vi "PowerModeSwitch.vi"(8 "error in (no error)":errorcluster, 11 "Data Cluster In":T1 {"VestaTemperature"."Water Heater Temp (°F)" min=32 max=203}) -> (0 "error out":errorcluster, 3 "Data Cluster out":T1 {"VestaTemperature"."Water Heater Temp (°F)" min=32 max=203}, 4 "Send_Vesta_Message":u8, 6 "Send_Timer_Message":u8)   [LabVIEW 2023]
uses:
  Drivers/Resideo Gas Valve/Type Definitions/Vesta Info.ctl
  Drivers/Resideo Gas Valve/Type Definitions/Temperature Control.ctl
  controls/Burner Duty Cycle.ctl
  controls/Timer Application Cluster.ctl
  controls/UI Data.ctl
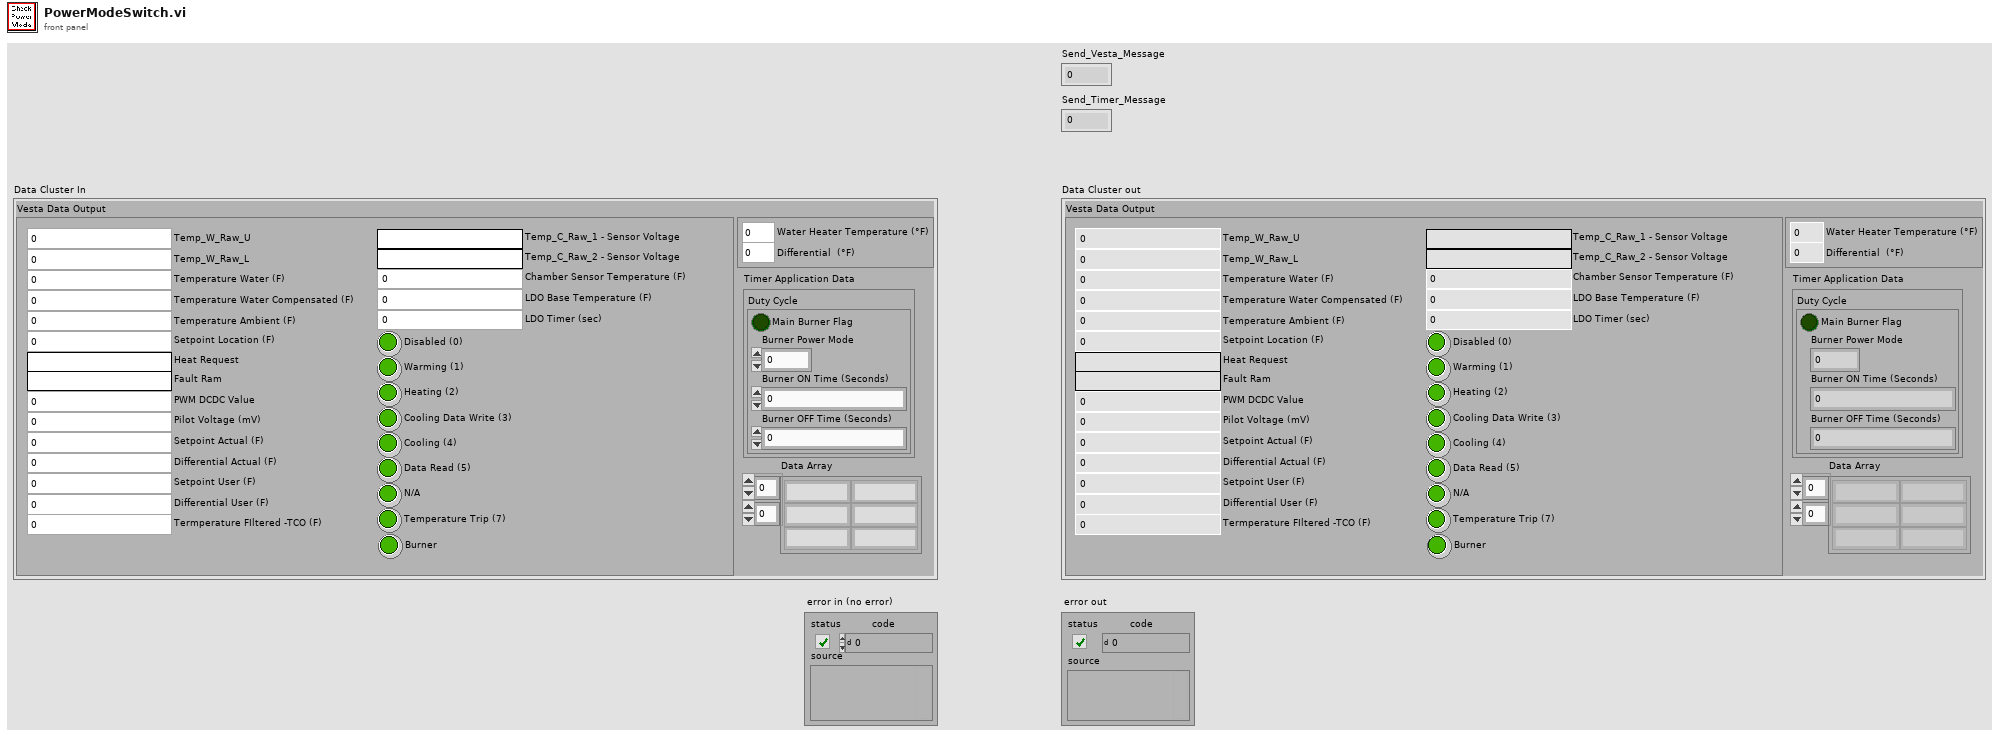
[diagram p1: front panel]
types:
  T1 = typedef "UI Data.ctl" = cluster{"Vesta Data Output":T2, "VestaTemperature":T3, "Timer Application Data":T4, "Data Array":string[][]}
  T2 = typedef "Vesta Info.ctl" = cluster{"Temp_W_Raw_U":u16, "Temp_W_Raw_L":u16, "Temperature Water (F)":dbl, "Temperature Water Compensated (F)":dbl, "Temperature Ambient (F)":dbl, "Setpoint Location (F)":dbl, "Heat Request":string, "Fault Ram":string, "PWM DCDC Value":u16, "Pilot Voltage (mV)":dbl, "Setpoint Actual (F)":dbl, "Differential Actual (F)":dbl, "Setpoint User (F)":dbl, "Differential User (F)":dbl, "Termperature FIltered -TCO (F)":dbl, "Temp_C_Raw_1 - Sensor Voltage":string, "Temp_C_Raw_2 - Sensor Voltage":string, "Chamber Sensor Temperature (F)":dbl, "LDO Base Temperature (F)":dbl, "LDO Timer (sec)":i16, "Disabled (0)":bool, "Warming (1)":bool, "Heating (2)":bool, "Cooling Data Write (3)":bool, "Cooling (4)":bool, "Data Read (5)":bool, "N/A":bool, "Temperature Trip (7)":bool, "Burner":bool}
  T3 = typedef "Temperature Control.ctl" = cluster{"Water Heater Temp (°F)":u16, "Differential  (°F)":dbl}
  T4 = typedef "Timer Application Cluster.ctl" = cluster{"Duty Cycle":T5}
  T5 = typedef "Burner Duty Cycle.ctl" = cluster{"Burner ON Time (Seconds)":dbl, "Burner OFF Time (Seconds)":dbl, "Main Burner Flag":bool, "Burner Power Mode":u8}
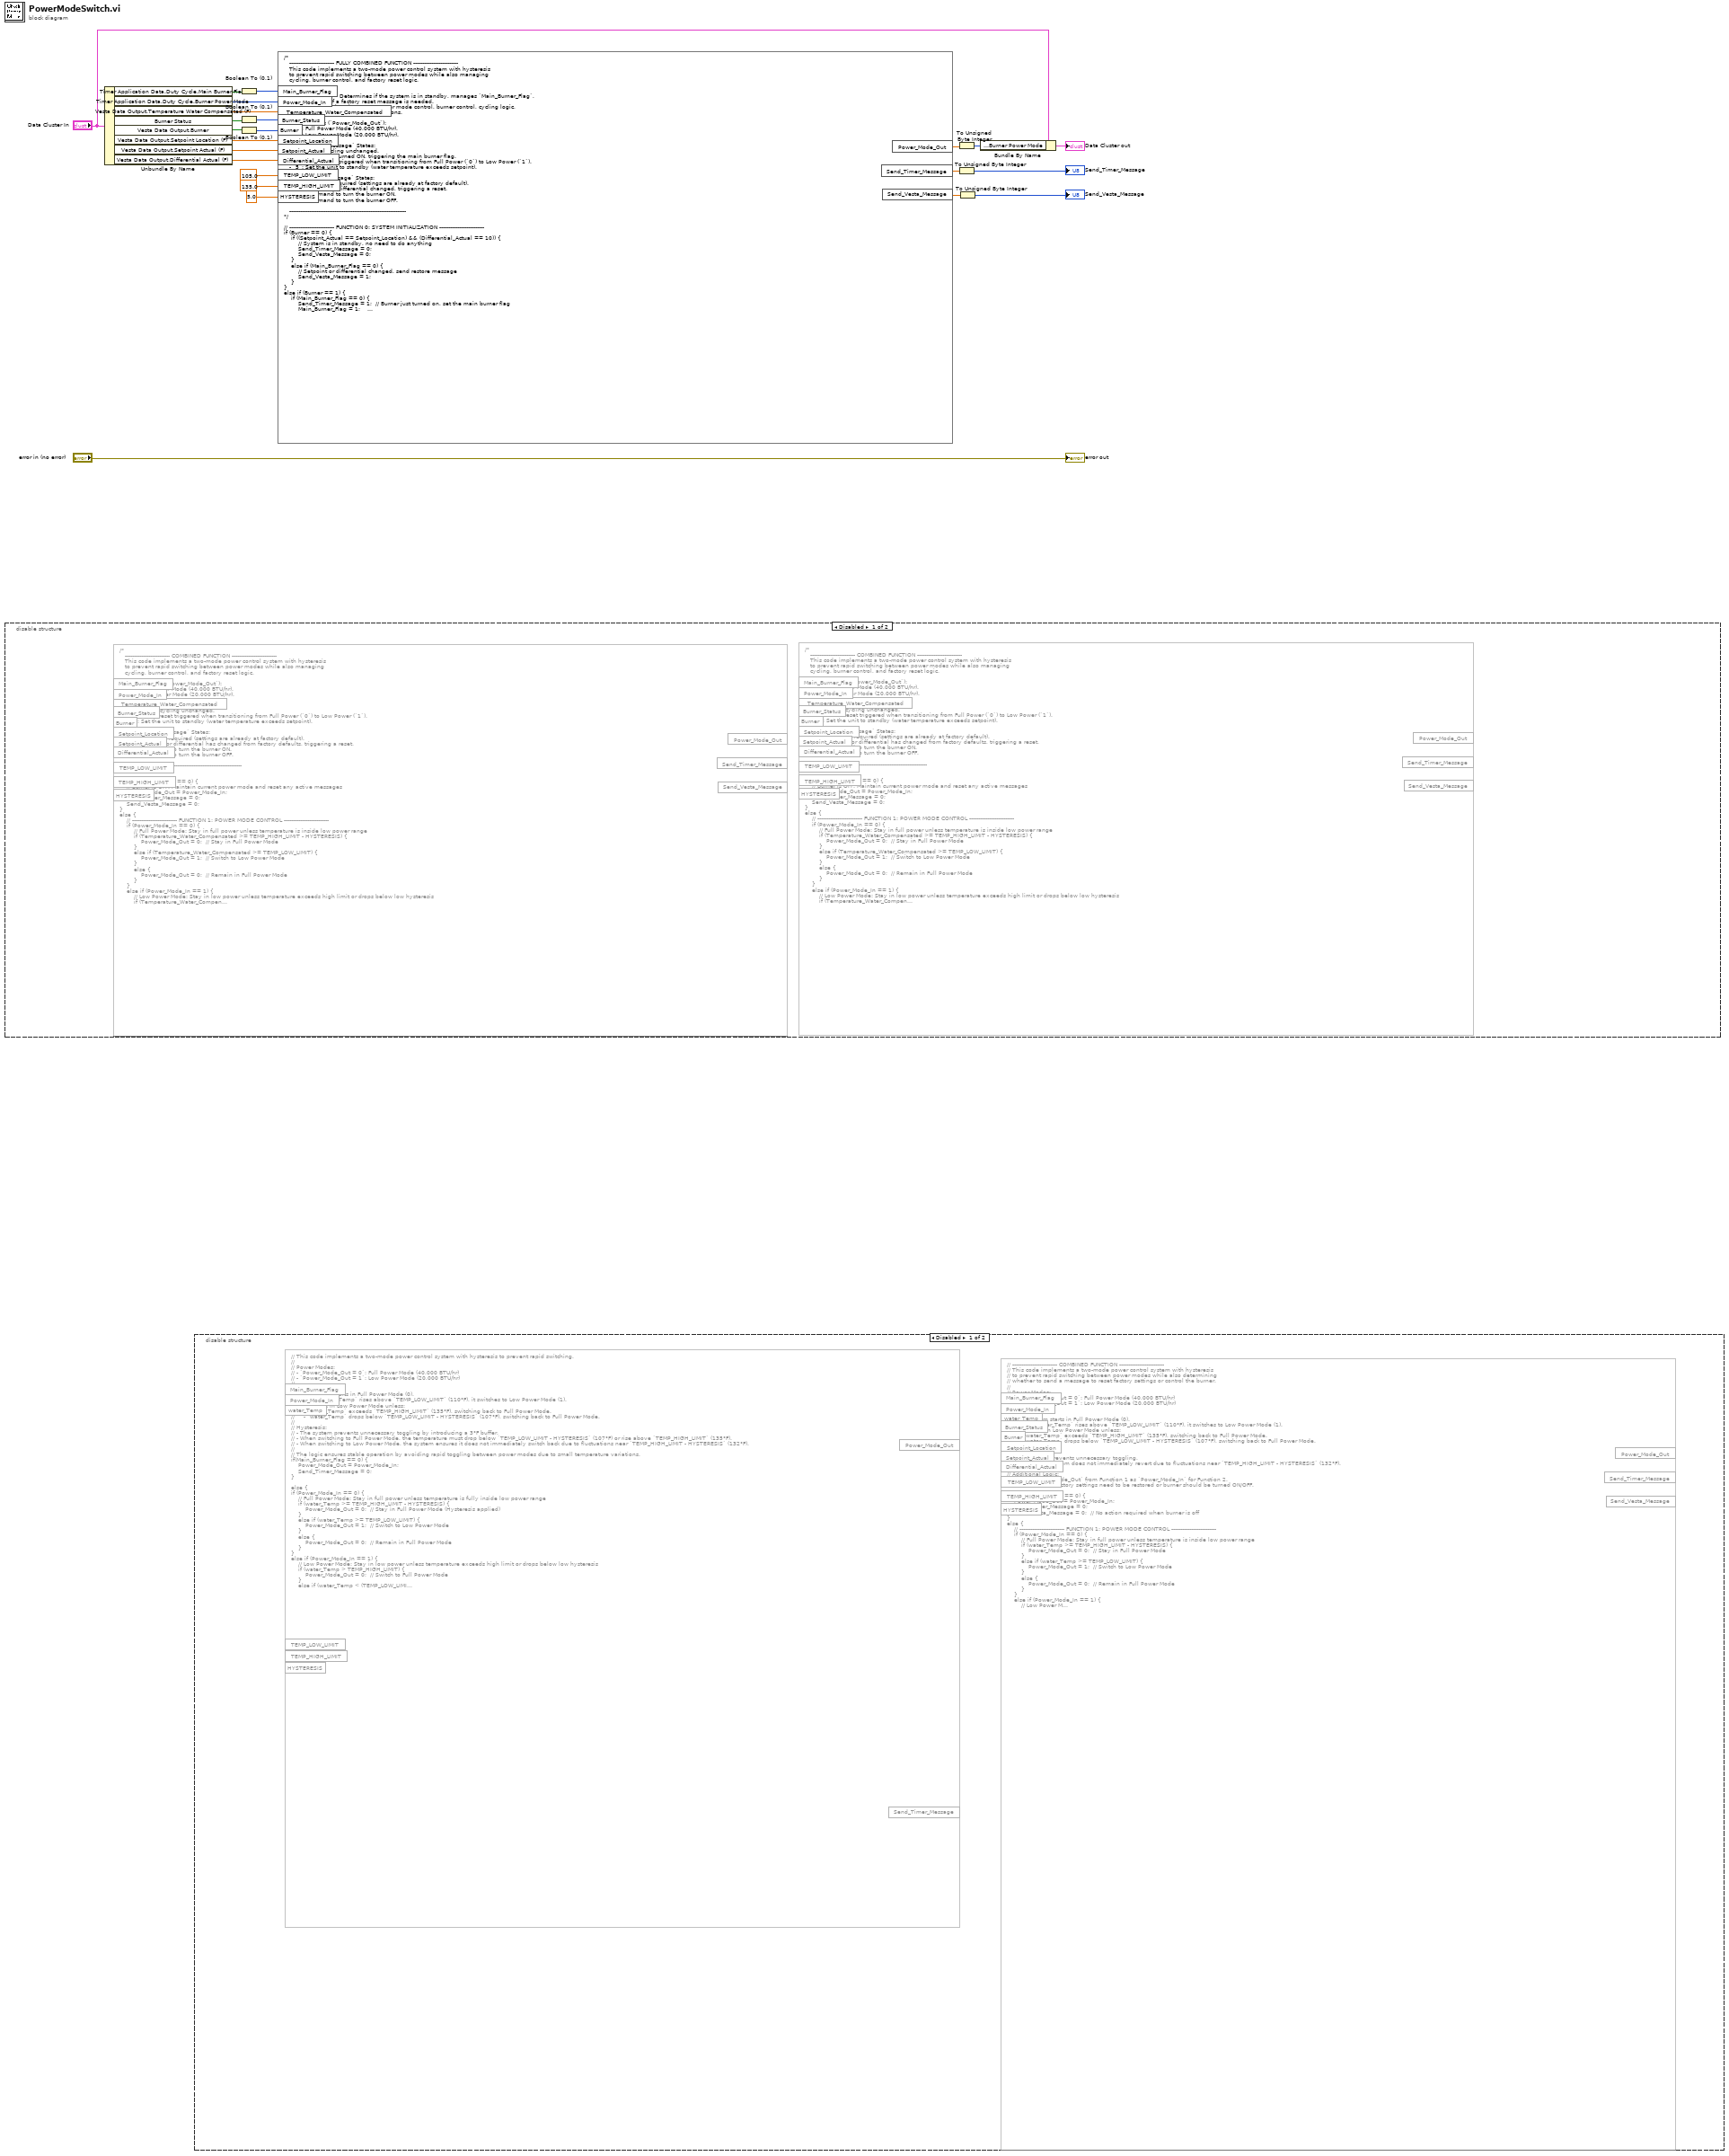
[diagram p0: block diagram]
diagram:
  n1 = disable-structure shown="Disabled" {
    frame Disabled {
      n2 = formula code="/*  \n   ------------------------- COMBINED FUNCTION -------------------------  \n   This code implements a two-mode power control system with hysteresis  \n   to prevent rapid switching between power modes while also managing  \n   cycling, burner control, and factory reset logic.\n\n   Power Modes (`Power_Mode_Out`):  \n   - `0`: Full Power Mode (40,000 BTU/hr).  \n   - `1`: Low Power Mode (20,000 BTU/hr).  \n\n   `Send_Timer_Message` States:  \n   - `0`: Leave cycling unchanged.  \n   - `2`: Timer reset triggered when transitioning from Full Power (`0`) to Low Power (`1`).  \n   - `5`: Set the unit to standby (water temperature exceeds setpoint).  \n\n   `Send_Vesta_Message` States:  \n   - `0`: No action required (settings are already at factory default).  \n   - `1`: Setpoint or differential has changed from factory defaults, triggering a reset.  \n   - `2`: Command to turn the burner ON.  \n   - `3`: Command to turn the burner OFF.  \n\n   -----------------------------------------------------------------\n*/\n\nif (Main_Burner_Flag == 0) {\n    // Burner is OFF: Maintain current power mode and reset any active messages\n    Power_Mode_Out = Power_Mode_In;\n    Send_Timer_Message = 0;\n    Send_Vesta_Message = 0;\n} \nelse {\n    // ------------------------- FUNCTION 1: POWER MODE CONTROL -------------------------\n    if (Power_Mode_In == 0) { \n        // Full Power Mode: Stay in full power unless temperature is inside low power range\n        if (Temperature_Water_Compensated >= TEMP_HIGH_LIMIT - HYSTERESIS) {\n            Power_Mode_Out = 0;  // Stay in Full Power Mode\n        } \n        else if (Temperature_Water_Compensated >= TEMP_LOW_LIMIT) {\n            Power_Mode_Out = 1;  // Switch to Low Power Mode\n        } \n        else {\n            Power_Mode_Out = 0;  // Remain in Full Power Mode\n        }\n    } \n    else if (Power_Mode_In == 1) { \n        // Low Power Mode: Stay in low power unless temperature exceeds high limit or drops below low hysteresis\n        if (Temperature_Water_Compensated > TEMP_HIGH_LIMIT) {\n            Power_Mode_Out = 0;  // Switch to Full Power Mode\n        } \n        else if (Temperature_Water_Compensated < (TEMP_LOW_LIMIT - HYSTERESIS)) {\n            Power_Mode_Out = 0;  // Switch to Full Power Mode\n        } \n        else {\n            Power_Mode_Out = 1;  // Stay in Low Power Mode\n        }\n    }\n\n    // Check if low power mode was just activated (Power_Mode_Out == 1).\n    if (Power_Mode_In == 0 && Power_Mode_Out == 1) { \n        Send_Timer_Message = 2; // Set reset flag\n    } \n    else { \n        Send_Timer_Message = 0; // Do not reset\n    }  \n\n    // ------------------------- FUNCTION 2: BURNER CONTROL -------------------------\n    if (Power_Mode_Out == 0) {  \n        // Check if the setpoint or differential has been altered from factory default.\n        if ((Setpoint_Actual != Setpoint_Location) || (Differential_Actual != 10)) {  \n            Send_Vesta_Message = 1;  // Command to restore default settings\n        }\n    } \n    else if (Power_Mode_Out == 1) {\n        // The timer routine determines when the burner should be ON or OFF.\n        if (Burner_Status == 1 && Burner == 0) {  \n            Send_Vesta_Message = 2;  // Command to turn the burner ON\n        }\n        if (Burner_Status == 0 && Burner == 1) {  \n            Send_Vesta_Message = 3;  // Command to turn the burner OFF\n        }\n    }\n\n    // ------------------------- FUNCTION 3: CYCLING CONTROL -------------------------\n    if (Temperature_Water_Compensated > Setpoint_Location) {\n        Send_Timer_Message = 5;  // Set the unit to standby\n    } \n\n    // ------------------------- FUNCTION 4: FACTORY RESET CHECK -------------------------\n    if (Temperature_Water_Compensated >= Setpoint_Location) {  \n        if ((Setpoint_Actual != Setpoint_Location) || (Differential_Actual != 10)) {  \n            if (Temperature_Water_Compensated != 0) {  \n                Send_Vesta_Message = 1;  // Send reset message\n            }\n        }\n    }\n}"() -> ()  [unwired: 11 in, 3 out]
      n3 = formula code="/*  \n   ------------------------- COMBINED FUNCTION -------------------------  \n   This code implements a two-mode power control system with hysteresis  \n   to prevent rapid switching between power modes while also managing  \n   cycling, burner control, and factory reset logic.\n\n   Power Modes (`Power_Mode_Out`):  \n   - `0`: Full Power Mode (40,000 BTU/hr).  \n   - `1`: Low Power Mode (20,000 BTU/hr).  \n\n   `Send_Timer_Message` States:  \n   - `0`: Leave cycling unchanged.  \n   - `2`: Timer reset triggered when transitioning from Full Power (`0`) to Low Power (`1`).  \n   - `5`: Set the unit to standby (water temperature exceeds setpoint).  \n\n   `Send_Vesta_Message` States:  \n   - `0`: No action required (settings are already at factory default).  \n   - `1`: Setpoint or differential has changed from factory defaults, triggering a reset.  \n   - `2`: Command to turn the burner ON.  \n   - `3`: Command to turn the burner OFF.  \n\n   -----------------------------------------------------------------\n*/\n\nif (Main_Burner_Flag == 0) {\n    // Burner is OFF: Maintain current power mode and reset any active messages\n    Power_Mode_Out = Power_Mode_In;\n    Send_Timer_Message = 0;\n    Send_Vesta_Message = 0;\n} \nelse {\n    // ------------------------- FUNCTION 1: POWER MODE CONTROL -------------------------\n    if (Power_Mode_In == 0) { \n        // Full Power Mode: Stay in full power unless temperature is inside low power range\n        if (Temperature_Water_Compensated >= TEMP_HIGH_LIMIT - HYSTERESIS) {\n            Power_Mode_Out = 0;  // Stay in Full Power Mode\n        } \n        else if (Temperature_Water_Compensated >= TEMP_LOW_LIMIT) {\n            Power_Mode_Out = 1;  // Switch to Low Power Mode\n        } \n        else {\n            Power_Mode_Out = 0;  // Remain in Full Power Mode\n        }\n    } \n    else if (Power_Mode_In == 1) { \n        // Low Power Mode: Stay in low power unless temperature exceeds high limit or drops below low hysteresis\n        if (Temperature_Water_Compensated > TEMP_HIGH_LIMIT) {\n            Power_Mode_Out = 0;  // Switch to Full Power Mode\n        } \n        else if (Temperature_Water_Compensated < (TEMP_LOW_LIMIT - HYSTERESIS)) {\n            Power_Mode_Out = 0;  // Switch to Full Power Mode\n        } \n        else {\n            Power_Mode_Out = 1;  // Stay in Low Power Mode\n        }\n    }\n\n    // Check if low power mode was just activated (Power_Mode_Out == 1).\n    if (Power_Mode_In == 0 && Power_Mode_Out == 1) { \n        Send_Timer_Message = 2; // Set reset flag\n    } \n    else { \n        Send_Timer_Message = 0; // Do not reset\n    }  \n\n    // ------------------------- FUNCTION 2: BURNER CONTROL -------------------------\n    if (Power_Mode_Out == 0) {  \n        // Check if the setpoint or differential has been altered from factory default.\n        if ((Setpoint_Actual != Setpoint_Location) || (Differential_Actual != 10)) {  \n            Send_Vesta_Message = 1;  // Command to restore default settings\n        }\n    } \n    else if (Power_Mode_Out == 1) {\n        // The timer routine determines when the burner should be ON or OFF.\n        if (Burner_Status == 1 && Burner == 0) {  \n            Send_Vesta_Message = 2;  // Command to turn the burner ON\n        }\n        if (Burner_Status == 0 && Burner == 1) {  \n            Send_Vesta_Message = 3;  // Command to turn the burner OFF\n        }\n    }\n\n    // ------------------------- FUNCTION 3: CYCLING CONTROL -------------------------\n    if (Temperature_Water_Compensated > Setpoint_Location) {\n        Send_Timer_Message = 5;  // Set the unit to standby\n    } \n\n    // ------------------------- FUNCTION 4: FACTORY RESET CHECK -------------------------\n    if (Temperature_Water_Compensated >= Setpoint_Location) {  \n        if ((Setpoint_Actual != Setpoint_Location) || (Differential_Actual != 10)) {  \n            if (Temperature_Water_Compensated != 0) {  \n                Send_Vesta_Message = 1;  // Send reset message\n            }\n        }\n    }\n}"() -> ()  [unwired: 11 in, 3 out]
    }
    frame Enabled {
    }
  }
  n4 = Unbundle By Name("Data Cluster In") -> ("Timer Application Data.Duty Cycle.Main Burner Flag"=w12:bool, "Timer Application Data.Duty Cycle.Burner Power Mode"=w17:u8, "Vesta Data Output.Temperature Water Compensated (F)"=w16:dbl, "Burner Status"=w10:bool, "Vesta Data Output.Burner"=w9:bool, "Vesta Data Output.Setpoint Location (F)"=w6:dbl, "Vesta Data Output.Setpoint Actual (F)"=w5:dbl, "Vesta Data Output.Differential Actual (F)"=w4:dbl)
  n5 = disable-structure shown="Disabled" {
    frame Disabled {
      n6 = formula code="// This code implements a two-mode power control system with hysteresis to prevent rapid switching.\n// \n// Power Modes:\n// - `Power_Mode_Out = 0`: Full Power Mode (40,000 BTU/hr)\n// - `Power_Mode_Out = 1`: Low Power Mode (20,000 BTU/hr)\n//\n// Behavior:\n// - The system starts in Full Power Mode (0).\n// - When `water_Temp` rises above `TEMP_LOW_LIMIT` (110°F), it switches to Low Power Mode (1).\n// - It remains in Low Power Mode unless:\n//     - `water_Temp` exceeds `TEMP_HIGH_LIMIT` (135°F), switching back to Full Power Mode.\n//     - `water_Temp` drops below `TEMP_LOW_LIMIT - HYSTERESIS` (107°F), switching back to Full Power Mode.\n//\n// Hysteresis:\n// - The system prevents unnecessary toggling by introducing a 3°F buffer.\n// - When switching to Full Power Mode, the temperature must drop below `TEMP_LOW_LIMIT - HYSTERESIS` (107°F) or rise above `TEMP_HIGH_LIMIT` (135°F).\n// - When switching to Low Power Mode, the system ensures it does not immediately switch back due to fluctuations near `TEMP_HIGH_LIMIT - HYSTERESIS` (132°F).\n//\n// The logic ensures stable operation by avoiding rapid toggling between power modes due to small temperature variations.\nif(Main_Burner_Flag == 0) {\n    Power_Mode_Out = Power_Mode_In;\n    Send_Timer_Message = 0;\n}\n\nelse {\nif (Power_Mode_In == 0) { \n    // Full Power Mode: Stay in full power unless temperature is fully inside low power range\n    if (water_Temp >= TEMP_HIGH_LIMIT - HYSTERESIS) {\n        Power_Mode_Out = 0;  // Stay in Full Power Mode (Hysteresis applied)\n    } \n    else if (water_Temp >= TEMP_LOW_LIMIT) {\n        Power_Mode_Out = 1;  // Switch to Low Power Mode\n    } \n    else {\n        Power_Mode_Out = 0;  // Remain in Full Power Mode\n    }\n} \nelse if (Power_Mode_In == 1) { \n    // Low Power Mode: Stay in low power unless temperature exceeds high limit or drops below low hysteresis\n    if (water_Temp > TEMP_HIGH_LIMIT) {\n        Power_Mode_Out = 0;  // Switch to Full Power Mode\n    } \n    else if (water_Temp < (TEMP_LOW_LIMIT - HYSTERESIS)) {\n        Power_Mode_Out = 0;  // Switch to Full Power Mode\n    } \n    else {\n        Power_Mode_Out = 1;  // Stay in Low Power Mode\n    }\n}\n\n // Check if low power mode was just activated (Power_Mode_Out == 1).\n// If so, trigger a timer reset.\nif (Power_Mode_In == 0 && Power_Mode_Out == 1  ) { \n        Send_Timer_Message = 2; // Set reset flag\n    } \nelse { \n        Send_Timer_Message = 0; // Do not reset\n    }  \n}"() -> ()  [unwired: 6 in, 2 out]
      n7 = formula code="// ------------------------- COMBINED FUNCTION -------------------------\n// This code implements a two-mode power control system with hysteresis\n// to prevent rapid switching between power modes while also determining \n// whether to send a message to reset factory settings or control the burner.\n//\n// Power Modes:\n// - `Power_Mode_Out = 0`: Full Power Mode (40,000 BTU/hr)\n// - `Power_Mode_Out = 1`: Low Power Mode (20,000 BTU/hr)\n//\n// Behavior:\n// - The system starts in Full Power Mode (0).\n// - When `water_Temp` rises above `TEMP_LOW_LIMIT` (110°F), it switches to Low Power Mode (1).\n// - It remains in Low Power Mode unless:\n//     - `water_Temp` exceeds `TEMP_HIGH_LIMIT` (135°F), switching back to Full Power Mode.\n//     - `water_Temp` drops below `TEMP_LOW_LIMIT - HYSTERESIS` (107°F), switching back to Full Power Mode.\n//\n// Hysteresis:\n// - A 3°F buffer prevents unnecessary toggling.\n// - Ensures the system does not immediately revert due to fluctuations near `TEMP_HIGH_LIMIT - HYSTERESIS` (132°F).\n//\n// Additional Logic:\n// - Uses `Power_Mode_Out` from Function 1 as `Power_Mode_In` for Function 2.\n// - Determines if factory settings need to be restored or burner should be turned ON/OFF.\n\nif (Main_Burner_Flag == 0) {\n    Power_Mode_Out = Power_Mode_In;\n    Send_Timer_Message = 0;\n    Send_Vesta_Message = 0;  // No action required when burner is off\n} \nelse {\n    // ------------------------- FUNCTION 1: POWER MODE CONTROL -------------------------\n    if (Power_Mode_In == 0) { \n        // Full Power Mode: Stay in full power unless temperature is inside low power range\n        if (water_Temp >= TEMP_HIGH_LIMIT - HYSTERESIS) {\n            Power_Mode_Out = 0;  // Stay in Full Power Mode\n        } \n        else if (water_Temp >= TEMP_LOW_LIMIT) {\n            Power_Mode_Out = 1;  // Switch to Low Power Mode\n        } \n        else {\n            Power_Mode_Out = 0;  // Remain in Full Power Mode\n        }\n    } \n    else if (Power_Mode_In == 1) { \n        // Low Power Mode: Stay in low power unless temperature exceeds high limit or drops below low hysteresis\n        if (water_Temp > TEMP_HIGH_LIMIT) {\n            Power_Mode_Out = 0;  // Switch to Full Power Mode\n        } \n        else if (water_Temp < (TEMP_LOW_LIMIT - HYSTERESIS)) {\n            Power_Mode_Out = 0;  // Switch to Full Power Mode\n        } \n        else {\n            Power_Mode_Out = 1;  // Stay in Low Power Mode\n        }\n    }\n\n    // Check if low power mode was just activated (Power_Mode_Out == 1).\n    if (Power_Mode_In == 0 && Power_Mode_Out == 1) { \n        Send_Timer_Message = 2; // Set reset flag\n    } \n    else { \n        Send_Timer_Message = 0; // Do not reset\n    }  \n\n    // ------------------------- FUNCTION 2: BURNER CONTROL -------------------------\n    if (Power_Mode_Out == 0) {  // Now using Power_Mode_Out as Power_Mode_In for function 2\n        // Check if the setpoint or differential has been altered from factory default.\n        if ((Setpoint_Actual != Setpoint_Location) || (Differential_Actual != 10)) {  \n            Send_Vesta_Message = 1;  // Command to restore default settings\n        }\n    } \n    else if (Power_Mode_Out == 1) {\n        // The timer routine determines when the burner should be ON or OFF.\n        // If the burner should be ON but is currently OFF, send a command to enable it.\n        if (Burner_Status == 1 && Burner == 0) {  \n            Send_Vesta_Message = 2;  // Command to turn the burner ON\n        }\n        // If the burner should be OFF but is currently ON, send a command to disable it.\n        if (Burner_Status == 0 && Burner == 1) {  \n            Send_Vesta_Message = 3;  // Command to turn the burner OFF\n        }\n    }\n}"() -> ()  [unwired: 11 in, 3 out]
    }
    frame Enabled {
    }
  }
  n8 = Boolean To (0,1)(Boolean=w12) -> (0, 1=w11:i16)
  n9 = Boolean To (0,1)(Boolean=w10) -> (0, 1=w8:i16)
  n10 = Boolean To (0,1)(Boolean=w9) -> (0, 1=w7:i16)
  n11 = formula code="/*  \n   ------------------------- FULLY COMBINED FUNCTION -------------------------  \n   This code implements a two-mode power control system with hysteresis  \n   to prevent rapid switching between power modes while also managing  \n   cycling, burner control, and factory reset logic.\n\n   Execution Order:  \n   1. **Function 0:** Determines if the system is in standby, manages `Main_Burner_Flag`,  \n      and decides if a factory reset message is needed.  \n   2. **Main Control Logic:** Runs power mode control, burner control, cycling logic,  \n      and checks for factory reset conditions.\n\n   Power Modes (`Power_Mode_Out`):  \n   - `0`: Full Power Mode (40,000 BTU/hr).  \n   - `1`: Low Power Mode (20,000 BTU/hr).  \n\n   `Send_Timer_Message` States:  \n   - `0`: Leave cycling unchanged.  \n   - `1`: Burner just turned ON, triggering the main burner flag.  \n   - `2`: Timer reset triggered when transitioning from Full Power (`0`) to Low Power (`1`).  \n   - `5`: Set the unit to standby (water temperature exceeds setpoint).  \n\n   `Send_Vesta_Message` States:  \n   - `0`: No action required (settings are already at factory default).  \n   - `1`: Setpoint or differential changed, triggering a reset.  \n   - `2`: Command to turn the burner ON.  \n   - `3`: Command to turn the burner OFF.  \n\n   -----------------------------------------------------------------\n*/\n\n// ------------------------- FUNCTION 0: SYSTEM INITIALIZATION -------------------------\nif (Burner == 0) {\n    if ((Setpoint_Actual == Setpoint_Location) && (Differential_Actual == 10)) {\n        // System is in standby, no need to do anything\n        Send_Timer_Message = 0;\n        Send_Vesta_Message = 0;\n    } \n    else if (Main_Burner_Flag == 0) {\n        // Setpoint or differential changed, send restore message\n        Send_Vesta_Message = 1;\n    }\n} \nelse if (Burner == 1) {\n    if (Main_Burner_Flag == 0) {\n        Send_Timer_Message = 1;  // Burner just turned on, set the main burner flag\n        Main_Burner_Flag = 1;    // Ensure the flag is updated before the main logic runs\n    } \n    else {\n        Send_Timer_Message = 0;  // Burner is already on, no need to re-trigger\n    }\n}\n\n// ------------------------- MAIN CONTROL LOGIC -------------------------\nif (Main_Burner_Flag == 0) {\n    // Burner is OFF: Maintain current power mode and reset any active messages\n    Power_Mode_Out = Power_Mode_In;\n    Send_Timer_Message = 0;\n    Send_Vesta_Message = 0;\n} \nelse {\n    // ------------------------- FUNCTION 1: POWER MODE CONTROL -------------------------\n    if (Power_Mode_In == 0) { \n        if (Temperature_Water_Compensated >= TEMP_HIGH_LIMIT - HYSTERESIS) {\n            Power_Mode_Out = 0;  // Stay in Full Power Mode\n        } \n        else if (Temperature_Water_Compensated >= TEMP_LOW_LIMIT) {\n            Power_Mode_Out = 1;  // Switch to Low Power Mode\n        } \n        else {\n            Power_Mode_Out = 0;  // Remain in Full Power Mode\n        }\n    } \n    else if (Power_Mode_In == 1) { \n        if (Temperature_Water_Compensated > TEMP_HIGH_LIMIT) {\n            Power_Mode_Out = 0;  // Switch to Full Power Mode\n        } \n        else if (Temperature_Water_Compensated < (TEMP_LOW_LIMIT - HYSTERESIS)) {\n            Power_Mode_Out = 0;  // Switch to Full Power Mode\n        } \n        else {\n            Power_Mode_Out = 1;  // Stay in Low Power Mode\n        }\n    }\n\n    // Check if low power mode was just activated (Power_Mode_Out == 1).\n    if (Power_Mode_In == 0 && Power_Mode_Out == 1) { \n        Send_Timer_Message = 2; // Set reset flag\n    }  \n\n    // ------------------------- FUNCTION 2: BURNER CONTROL -------------------------\n    if (Power_Mode_Out == 0) {  \n        if ((Setpoint_Actual != Setpoint_Location) || (Differential_Actual != 10)) {  \n            Send_Vesta_Message = 1;  // Command to restore default settings\n        }\n    } \n    else if (Power_Mode_Out == 1) {\n        if (Burner_Status == 1 && Burner == 0) {  \n            Send_Vesta_Message = 2;  // Command to turn the burner ON\n        }\n        if (Burner_Status == 0 && Burner == 1) {  \n            Send_Vesta_Message = 3;  // Command to turn the burner OFF\n        }\n    }\n\n    // ------------------------- FUNCTION 3: CYCLING CONTROL -------------------------\n    if (Temperature_Water_Compensated > Setpoint_Location) {\n        Send_Timer_Message = 5;  // Set the unit to standby\n    } \n\n    // ------------------------- FUNCTION 4: FACTORY RESET CHECK -------------------------\n    if (Temperature_Water_Compensated >= Setpoint_Location) {  \n        if ((Setpoint_Actual != Setpoint_Location) || (Differential_Actual != 10)) {  \n            if (Temperature_Water_Compensated != 0) {  \n                Send_Vesta_Message = 1;  // Send reset message\n            }\n        }\n    }\n}"("Temperature_Water_Compensated"=w16, "Power_Mode_In"=w17, "TEMP_LOW_LIMIT"=105.0 ("input variable"), "TEMP_HIGH_LIMIT"=135.0 ("input variable"), "HYSTERESIS"=5.0 ("input variable"), "Main_Burner_Flag"=w11, "Burner_Status"=w8, "Burner"=w7, "Setpoint_Location"=w6, "Setpoint_Actual"=w5, "Differential_Actual"=w4) -> ("Power_Mode_Out"=w20:dbl, "Send_Timer_Message"=w18:dbl, "Send_Vesta_Message"=w2:dbl)
  n12 = To Unsigned Byte Integer(number=w20) -> (unsigned 8bit integer=w13:u8)
  n13 = To Unsigned Byte Integer(number=w18) -> (unsigned 8bit integer=→"Send_Timer_Message":u8)
  n14 = To Unsigned Byte Integer(number=w2) -> (unsigned 8bit integer=→"Send_Vesta_Message":u8)
  n15 = Bundle By Name(cluster="Data Cluster In", "Timer Application Data.Duty Cycle.Burner Power Mode"=w13) -> (→"Data Cluster out":T1)
  "error out" <- "error in (no error)"
